vi "Edit-GUI-param-defaults-with-dialog.vi"() -> ()   [LabVIEW 2013, in "CameraVision.lvlib" / "CV-Main.lvclass"]
uses:
  CV-Main.lvclass
  UI/Parameters-gui.ctl
  Configuration/Configuration-parameters-gui.ctl
  Acquisition/Acquisition-parameters-gui.ctl
  Acquisition/Trigger-modes.ctl
  Acquisition/Exposure-modes.ctl
  Storage/Storage-parameters-gui.ctl
  Storage/Storage-types.ctl
  Correction/Correction-parameters-gui.ctl
  Correction/Smoothing.ctl
  Correction/Background-correction.ctl
  Analysis/Analysis-parameters-gui.ctl
  Temperature/Temperature-parameters-gui.ctl
  Mapping/Mapping-parameters-gui.ctl
  Mapping/Mapping-characteristic.ctl
  Filter/Filter-parameters-gui.ctl
  Filter/Filter-settings.ctl
  Filter/Filter-characteristic.ctl
  Filter/Filter-apply.ctl
  <vilib>/Utility/xml.llb/Write to XML File(string).vi
  UI/CV-UI.lvclass
  Storage/CV-Storage.lvclass
  Acquisition/CV-Acquisition.lvclass
  Configuration/CV-Configuration.lvclass
  Correction/CV-Correction.lvclass
  Analysis/CV-Analysis.lvclass
  Temperature/CV-Temperature.lvclass
  Mapping/CV-Mapping.lvclass
  Filter/CV-Filter.lvclass
panel:
  in  "Relative save path":string="Program data\\parameters-gui.xml"
  in  "Parameters":T1={"Configuration params"={"Number of cameras"=1, "Camera 1 port"=enum."A", "ROI width"=1248, "ROI height"=1082, "Reset ROI"=FALSE, "Width scale"=0.05, "Height scale"=0.05, "Center Y cam. 1"=541, "Center X cam. 1"=624, "Center Y cam. 2"=541, "Center X cam. 2"=624}, "Acquisition params"={"Acquisition mode"=enum."Continuous batch", "Batch size"=50, "Image buffer size"=10, "Trigger mode"=enum."Framegrabber timed (sync.)", "Duration HH"=1.0, "Acquisition start"=enum."Immediate", "Duration SS"=0.01, "Duration MM"=0.01, "Start time"=timestamp(0 s since 1904-01-01), "Max. frame rate"=5.0, "Exposure time cam. 1"=1.0, "Exposure time cam. 2"=1.0, "Exposure mode"=enum."Linear", "Value 1"=17.0, "Value 2"=14.0, "Time 1"=1000.0, "Time 2"=1000.0}, "Storage params"={"Base file name"="Test", "Storage directory"=path "C:/CameraVision/Results", "Save what?"={"Original"=FALSE, "Corrected"=FALSE, "Binary"=FALSE, "Temperature"=FALSE, "Characteristics"=FALSE, "Mapping"=FALSE, "TemperatureValues"=FALSE}, "Image file type"=enum."BMP", "Comments"="", "Storage mode"=enum."1 file for all layers ", "Start iteration/layer"=0}, "Correction params"={"Background correction"=FALSE, "Hot-pixel correction"=FALSE, "Black image cam. 1"=path "C:/CameraVision/Black images/Black-CameraA-Full.bmp", "Black image cam. 2"=path "C:/CameraVision/Black images/Black-CameraB-Full.bmp", "Y-shift"=0, "X-shift"=1, "Correlation algorithm"=enum."Fixed shift", "Noise treshold"=40.0, "Smoothing algorithm"=enum."Noise tresholding", "2nd image correlation"=FALSE, "Image smoothing"=FALSE, "Background correction method"=enum."Hardware"}, "Analysis params"={"Binarization treshold"=120.0, "Image characteristics"=FALSE, "Melt-pool characteristics"=FALSE}, "Temperature params"={"Temperature field"=FALSE, "Ratio correction factor"=1.0, "Temperature value"=FALSE, "Y-coord."=40.0, "X-coord."=0.0, "Averaging center"=enum."Fixed coordinates (pixel)", "Averaging shape"=enum."Point", "Minor axis"=0.0, "Major axis"=0.0}, "Mapping params"={"Enable mapping"=FALSE, "Automatic timing"=FALSE, "Scan pattern file"=path "C:/CameraVision/Scan patterns/Template.sp", "Start off-set"=0.0, "Default map characteristic"=enum."Average intensity [0-255]", "Default mark speed"=1000, "Jump speed"=1000}, "Filter params"={"Filter array"=[], "Storage filters"={"Filter images"=FALSE, "Filter characteristics"=FALSE, "Filter temperature"=FALSE}}} {"Mapping params"."Jump speed" min=1; "Mapping params"."Default mark speed" min=1; "Mapping params"."Start off-set" step=0.0001; "Temperature params"."Major axis" min=0.0; "Temperature params"."Minor axis" min=0.0; "Temperature params"."Ratio correction factor" min=0.0 step=0.0001 format="%#.4g"; "Analysis params"."Binarization treshold" min=0 max=255 step=1; "Correction params"."Noise treshold" min=0 max=255 step=1; "Configuration params"."Center X cam. 2" min=4 max=1244 step=8; "Configuration params"."Center Y cam. 2" min=1 max=1082 step=1; "Configuration params"."Center X cam. 1" min=4 max=1244 step=8; "Configuration params"."Center Y cam. 1" min=1 max=1082 step=1; "Configuration params"."Height scale" min=0.001 step=0.001 format="%.3f"; "Configuration params"."Width scale" min=0.001 step=0.001 format="%.3f"; "Configuration params"."Number of cameras" min=1 max=2 step=1; "Configuration params"."ROI width" min=8 max=1248 step=8; "Configuration params"."ROI height" min=1 max=1082 step=1; "Acquisition params"."Exposure time cam. 2" min=0.01 step=0.01 format="%#.2g"; "Acquisition params"."Exposure time cam. 1" min=0.01 step=0.01 format="%#.2g"; "Acquisition params"."Max. frame rate" min=0.0001 max=1000000.0 format="%#.4g"; "Acquisition params"."Start time" format="%<%X\n%x>T"; "Acquisition params"."Duration MM" min=0 max=59 step=1 format="%02.0f"; "Acquisition params"."Duration SS" min=0 max=59 step=1 format="%02.0f"; "Acquisition params"."Duration HH" min=0 step=1 format="%02.0f"; "Acquisition params"."Image buffer size" min=1 max=10000 step=1 format="%#.0f"; "Acquisition params"."Batch size" min=1 max=50000 step=1}
  in  "Cancel":bool
  in  "OK":bool
  # ":"
  # ":"
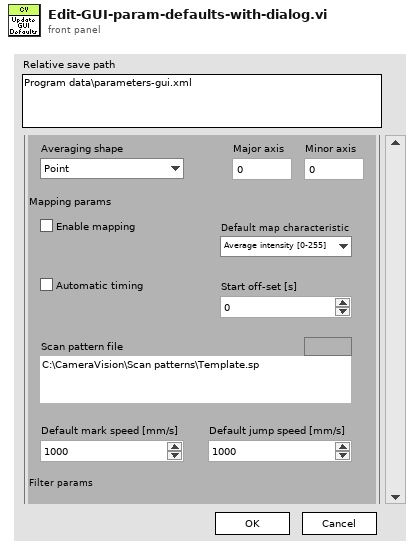
[diagram p1: front panel]
types:
  T1 = typedef "CameraVision.lvlib/CV-UI.lvclass/Parameters-gui.ctl" = cluster{"Configuration params":T2, "Acquisition params":T3, "Storage params":T6, "Correction params":T8, "Analysis params":T11, "Temperature params":T12, "Mapping params":T13, "Filter params":T15}
  T2 = typedef "CameraVision.lvlib/CV-Configuration.lvclass/Configuration-parameters-gui.ctl" = cluster{"Number of cameras":i32, "Camera 1 port":enum16{"A", "B"}, "ROI width":u32, "ROI height":u32, "Reset ROI":bool, "Width scale":dbl, "Height scale":dbl, "Center Y cam. 1":i32, "Center X cam. 1":i32, "Center Y cam. 2":i32, "Center X cam. 2":i32}
  T3 = typedef "CameraVision.lvlib/CV-Acquisition.lvclass/Acquisition-parameters-gui.ctl" = cluster{"Acquisition mode":enum16{"Continuous", "Continuous batch", "Single batch", "Single batch -delayed"}, "Batch size":i32, "Image buffer size":i32, "Trigger mode":T4, "Duration HH":sgl, "Acquisition start":enum16{"Immediate", "Post-phoned"}, "Duration SS":sgl, "Duration MM":sgl, "Start time":timestamp, "Max. frame rate":dbl, "Exposure time cam. 1":dbl, "Exposure time cam. 2":dbl, "Exposure mode":T5, "Value 1":dbl, "Value 2":dbl, "Time 1":dbl, "Time 2":dbl}
  T4 = typedef "CameraVision.lvlib/CV-Acquisition.lvclass/Trigger-modes.ctl" = enum16{"Camera timed (not sync.)", "Framegrabber timed (sync.)", "Software timed (sync.)", "External timing (sync.)", "Manual (sync.)", "Gated - camera (not sync.)", "Gated - grabber (sync.)", "Gated - software (sync.)", "Gated - external (sync.)"}
  T5 = typedef "CameraVision.lvlib/CV-Acquisition.lvclass/Exposure-modes.ctl" = enum16{"Linear", "LinLog"}
  T6 = typedef "CameraVision.lvlib/CV-Storage.lvclass/Storage-parameters-gui.ctl" = cluster{"Base file name":string, "Storage directory":path, "Save what?":T7, "Image file type":enum16{"JPG", "BMP", "PNG"}, "Comments":string, "Storage mode":enum16{"1 file per layer", "1 file for all layers "}, "Start iteration/layer":u16}
  T7 = typedef "CameraVision.lvlib/CV-Storage.lvclass/Storage-types.ctl" = cluster{"Original":bool, "Corrected":bool, "Binary":bool, "Temperature":bool, "Characteristics":bool, "Mapping":bool, "TemperatureValues":bool}
  T8 = typedef "CameraVision.lvlib/CV-Correction.lvclass/Correction-parameters-gui.ctl" = cluster{"Background correction":bool, "Hot-pixel correction":bool, "Black image cam. 1":path, "Black image cam. 2":path, "Y-shift":i32, "X-shift":i32, "Correlation algorithm":enum16{"Fixed shift", "Cross-correlation", "Cross-correlation (5steps)", "Melt-pool center"}, "Noise treshold":sgl, "Smoothing algorithm":T9, "2nd image correlation":bool, "Image smoothing":bool, "Background correction method":T10}
  T9 = typedef "CameraVision.lvlib/CV-Correction.lvclass/Smoothing.ctl" = enum16{"Noise tresholding", "NT+Median filter", "NT+Gaussian filter"}
  T10 = typedef "CameraVision.lvlib/CV-Correction.lvclass/Background-correction.ctl" = enum16{"Hardware", "Software"}
  T11 = typedef "CameraVision.lvlib/CV-Analysis.lvclass/Analysis-parameters-gui.ctl" = cluster{"Binarization treshold":sgl, "Image characteristics":bool, "Melt-pool characteristics":bool}
  T12 = typedef "CameraVision.lvlib/CV-Temperature.lvclass/Temperature-parameters-gui.ctl" = cluster{"Temperature field":bool, "Ratio correction factor":dbl, "Temperature value":bool, "Y-coord.":dbl, "X-coord.":dbl, "Averaging center":enum16{"Fixed coordinates (pixel)", "Fixed coordinates (mm)", "Melt-pool center"}, "Averaging shape":enum16{"Point", "Circle", "Ellipse"}, "Minor axis":dbl, "Major axis":dbl}
  T13 = typedef "CameraVision.lvlib/CV-Mapping.lvclass/Mapping-parameters-gui.ctl" = cluster{"Enable mapping":bool, "Automatic timing":bool, "Scan pattern file":path, "Start off-set":dbl, "Default map characteristic":T14, "Default mark speed":i32, "Jump speed":i32}
  T14 = typedef "CameraVision.lvlib/CV-Mapping.lvclass/Mapping-characteristic.ctl" = enum16{"Average intensity [0-255]", "Peak intensity [0-255]", "Melt-pool size [mm²]", "Melt-pool aspect ratio []", "Melt-pool fragments []", "Average temperature [°C]", "Max. temperature [°C]", "Min. temperature [°C]", "Std. dev. temperature [°C]"}
  T15 = typedef "CameraVision.lvlib/CV-Filter.lvclass/Filter-parameters-gui.ctl" = cluster{"Filter array":T16[], "Storage filters":T18}
  T16 = typedef "CameraVision.lvlib/CV-Filter.lvclass/Filter-settings.ctl" = cluster{"Characteristic":T17, "Monitor":bool, "Min.":dbl, "Max.":dbl, "Min. Thres.":dbl, "Min. Dur.":u16, "Report":bool}
  T17 = typedef "CameraVision.lvlib/CV-Filter.lvclass/Filter-characteristic.ctl" = enum16{"Average intensity [0-255]", "Peak intensity [0-255]", "Melt-pool size [mm²]", "Melt-pool aspect ratio []", "Melt-pool fragments []", "Melt-pool position X [pixel]", "Melt-pool position Y [pixel]", "Average temperature [°C]", "Max. temperature [°C]", "Min. temperature [°C]", "Std. dev. temperature [°C]"}
  T18 = typedef "CameraVision.lvlib/CV-Filter.lvclass/Filter-apply.ctl" = cluster{"Filter images":bool, "Filter characteristics":bool, "Filter temperature":bool}
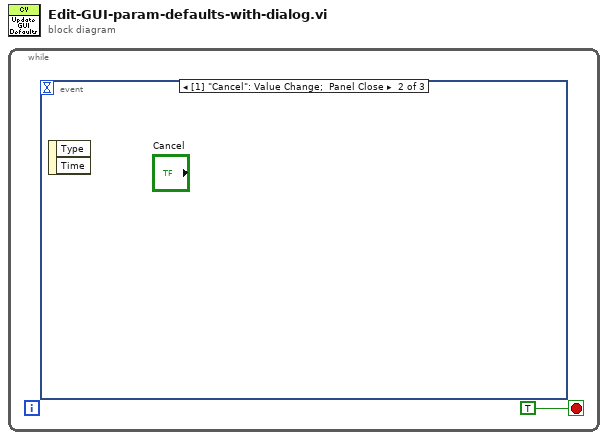
[diagram p0: block diagram]
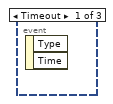
[diagram p2: hidden frame]
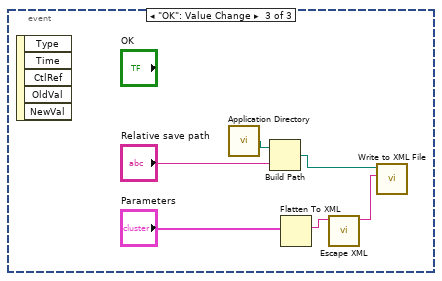
[diagram p3: hidden frame]
diagram:
  n1 = while {
    stop <- TRUE stop-if-true
    n2 = event shown="[1] \"Cancel\": Value Change;  Panel Close" {
      selector: _ -> [_ _ _]
      dyn-events: _ -> [_ _ _]
      timeout: _ -> [_ _ _]
      event Timeout {
        n3 = event-data() -> ()  [unwired: 1 in, 2 out]
      }
      event "Cancel": Value Change; Panel Close {
        n4 = event-data() -> ()  [unwired: 1 in, 2 out]
      }
      event "OK": Value Change {
        n5 = event-data() -> ()  [unwired: 1 in, 5 out]
        n6 = call <vilib>:"Application Directory.vi"() -> ("Application Directory"=w3:path)
        n7 = Build Path(base path=w3, name or relative path="Relative save path") -> (appended path=w6:path)
        n8 = Flatten To XML(anything="Parameters") -> (xml string=w4:string)
        n9 = call <vilib>:"Escape XML.vi"("XML String In"=w4) -> ("XML String Out"=w7:string)  [unwired: 9 in, 1 out]
        n10 = call-poly <vilib>:"Write to XML File.vi"("XML Input"=w7, "XML File Path"=w6) -> ()  [unwired: 7 in, 3 out]
      }
    }
  }
